vi "Generate Noisy Ringdowns.vi"(8 "error in":errorcluster, 9 "Ramp Pattern":dbl[](array[numeric]), 10 "ExpData In":cluster{"A":dbl, "B":dbl, "tau":dbl}[](array[cluster]), 11 "Filter":bool) -> (0 "error out":errorcluster, 3 "RD Data Out":dbl[][](array[numeric]))   [LabVIEW 2015, in "CRDS.lvclass"]
uses:
  Main/CRDS.lvclass
  General/Math/Fit Exponential Class/Fit Exponential.lvclass
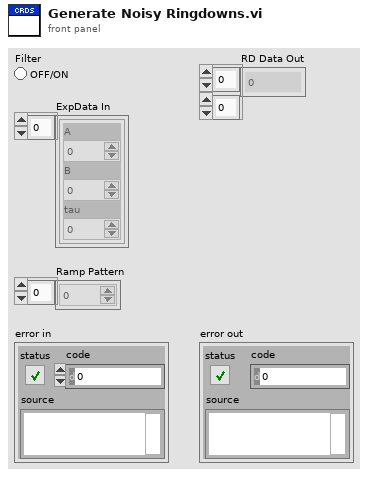
[diagram p1: front panel]
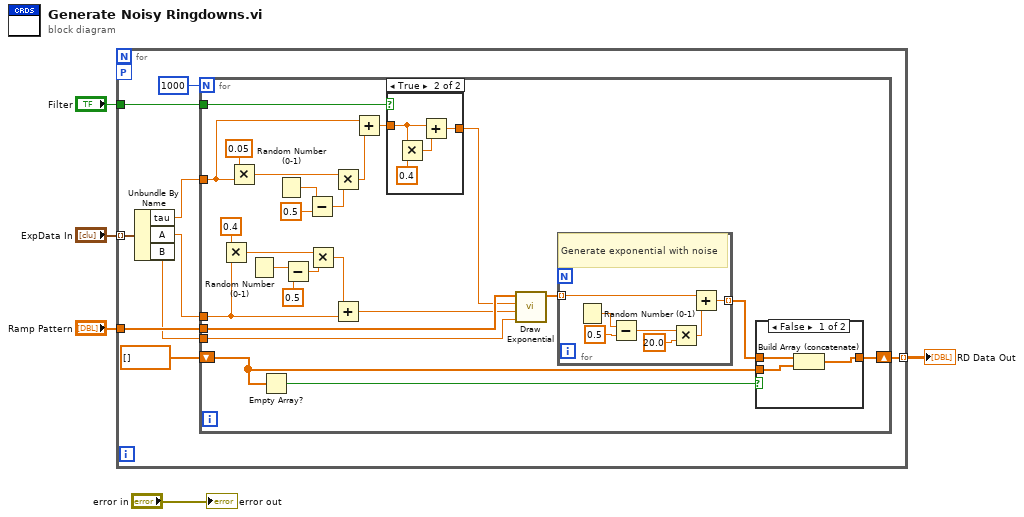
[diagram p0: block diagram]
diagram:
  n1 = for {
    tunnel: "Ramp Pattern" -> [w14]
    tunnel: [w11] -> w3 mode=indexing
    workers-P: _ -> [_]
    tunnel: "Filter" -> [w10]
    tunnel: "ExpData In" -> [w9] mode=indexing
    n2 = Unbundle By Name(w9) -> ("tau"=w8:dbl, "A"=w7:dbl, "B"=w6:dbl)
    n3 = for {
      N: 1000 -> [_]
      tunnel: w14 -> [w39]
      shift-right: [w35] -> w11
      shift-left: dbl[] [] -> [w34]
      tunnel: w8 -> [w27]
      tunnel: w7 -> [w20]
      tunnel: w10 -> [w18]
      tunnel: w6 -> [w15]
      n4 = Multiply(x=0.4 ("y"), y=w20) -> (x*y=w25:dbl)
      n5 = Multiply(x=0.05 ("y"), y=w27) -> (x*y=w30:dbl)
      n6 = Random Number (0-1)() -> (number: 0 to 1=w23:dbl)
      n7 = Empty Array?(array=w34) -> (empty?=w37:bool)
      n8 = Random Number (0-1)() -> (number: 0 to 1=w32:dbl)
      n9 = Subtract(x=w23, y=0.5) -> (x-y=w22:dbl)
      n10 = Subtract(x=w32, y=0.5) -> (x-y=w29:dbl)
      n11 = Multiply(x=w25, y=w22) -> (x*y=w21:dbl)
      n12 = Multiply(x=w30, y=w29) -> (x*y=w28:dbl)
      n13 = Add(x=w21, y=w20) -> (x+y=w19:dbl)
      n14 = Add(x=w27, y=w28) -> (x+y=w17:dbl)
      n15 = case shown="True" w18 {
        tunnel: w17 -> [w40 w42]
        tunnel: [w40 w41] -> w16
        frame False {
        }
        frame True {
          n16 = Multiply(x=w42, y=0.4) -> (x*y=w43:dbl)
          n17 = Add(x=w42, y=w43) -> (x+y=w41:dbl)
        }
      }
      n18 = call "Draw Exponential.vi"("B"=w15, "A"=w19, "tau"=w16, "time"=w39) -> ("ExponentialOut"=w38:dbl[])  [unwired: 7 in]
      n19 = for {
        tunnel: w38 -> [w50] mode=indexing
        tunnel: [w49] -> w36 mode=indexing
        # "Generate exponential with noise"
        n20 = Random Number (0-1)() -> (number: 0 to 1=w55:dbl)
        n21 = Subtract(x=w55, y=0.5) -> (x-y=w53:dbl)
        n22 = Multiply(x=w53, y=20.0) -> (x*y=w51:dbl)
        n23 = Add(x=w50, y=w51) -> (x+y=w49:dbl)
      }
      n24 = case shown="False" w37 {
        tunnel: w36 -> [w47 w48]
        tunnel: [w45 w48] -> w35
        tunnel: w34 -> [w46 _]
        frame False {
          n25 = Build Array (concatenate)(w47, w46) -> (w45:dbl[])
        }
        frame True {
        }
      }
    }
  }
  "RD Data Out" <- w3
  "error out" <- "error in"
